vi "Convert Variant Data to String.vi"(8 "error in":errorcluster, 11 "Data":variant[][](array[variant])=array196x32[6272 elements]) -> (0 "error out":errorcluster, 3 "Data":string[][](array[string]))   [LabVIEW 2019, in "Simple SysDef API.lvlib"]
uses:
  <userlib>/SimpleSysDef/Simple SysDef API.lvlib
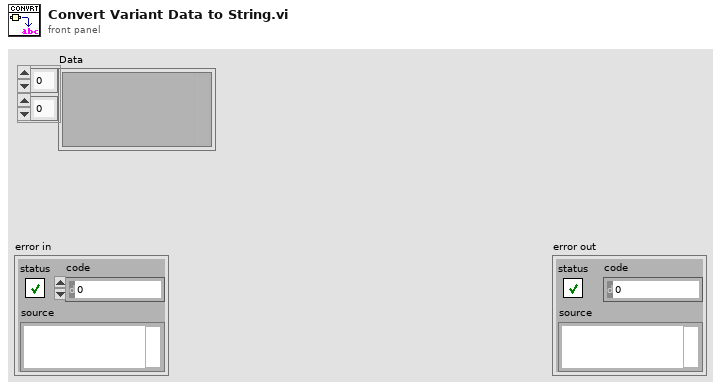
[diagram p1: front panel]
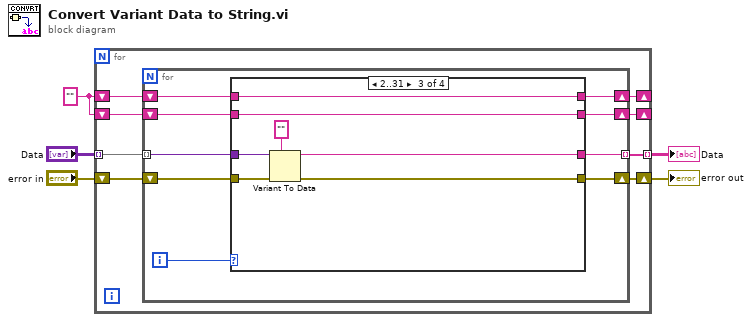
[diagram p0: block diagram]
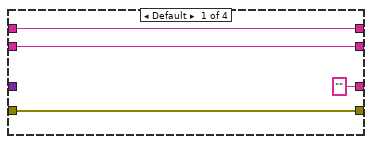
[diagram p2: hidden frame]
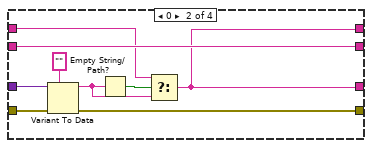
[diagram p3: hidden frame]
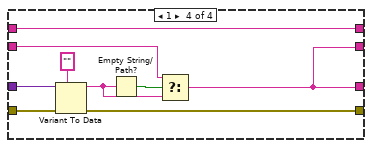
[diagram p4: hidden frame]
diagram:
  w1 = "" ("Format String (optional)")
  n1 = for {
    tunnel: "Data" -> [w13] mode=indexing
    tunnel: [w12] -> w4 mode=indexing
    shift-right: [w11] -> w2
    shift-left: "error in" -> [w10]
    shift-right: [w9] -> _
    shift-left: w1 -> [w8]
    shift-right: [w7] -> _
    shift-left: w1 -> [w6]
    n2 = for {
      tunnel: w13 -> [w22] mode=indexing
      tunnel: [w21] -> w12 mode=indexing
      shift-right: [w20] -> w11
      shift-left: w10 -> [w19]
      shift-right: [w17] -> w9
      shift-left: w8 -> [w16]
      shift-right: [w15] -> w7
      shift-left: w6 -> [w14]
      i -> [w18]
      n3 = case shown="2..31" w18 {
        tunnel: w22 -> [_ w35 w42 w51]
        tunnel: ["" ("Format String (optional)") w27 w37 w43] -> w21
        tunnel: [w26 w33 w40 w49] -> w20
        tunnel: w19 -> [w26 w32 w39 w48]
        tunnel: [w23 w27 w36 w47] -> w17
        tunnel: w16 -> [w23 w29 w36 w47]
        tunnel: [w24 w31 w38 w43] -> w15
        tunnel: w14 -> [w24 w31 w38 w45]
        frame Default {
        }
        frame 0 {
          n4 = Variant To Data(error in=w32, type="" ("Format String (optional)"), Variant=w35) -> (data=w28:string, error out=w33:errorcluster)
          n5 = Empty String/Path?(string/path=w28) -> (empty?=w30:bool)
          n6 = Select(t=w29, s=w30, f=w28) -> (s? t:f=w27:string)
        }
        frame 2..31 {
          n7 = Variant To Data(error in=w39, type="" ("Format String (optional)"), Variant=w42) -> (data=w37:string, error out=w40:errorcluster)
        }
        frame 1 {
          n8 = Variant To Data(error in=w48, type="" ("Format String (optional)"), Variant=w51) -> (data=w44:string, error out=w49:errorcluster)
          n9 = Empty String/Path?(string/path=w44) -> (empty?=w46:bool)
          n10 = Select(t=w45, s=w46, f=w44) -> (s? t:f=w43:string)
        }
      }
    }
  }
  "Data" <- w4
  "error out" <- w2
